vi "G#MethodTemplates_GetAttributes.vi"(0 "reference in":refnum<class "G#MethodTemplates.lvclass">, 1 "return data? (T)":bool=TRUE, 5 "error in (no error)":errorcluster) -> (14 "reference out":refnum<class "G#MethodTemplates.lvclass">, 15 "attributes ref":T2, 16 "attributes":T1, 19 "error out":errorcluster)   [LabVIEW 2020, in "G#MethodTemplates.lvclass"]
doc: "Returns a reference and if wanted the actual data values of the attributes. This method is used by the subclasses to access parent attributes."
uses:
  G#MethodTemplates.lvclass
  ObjectAttributesRef.ctl
  protected/ObjectAttributes.ctl
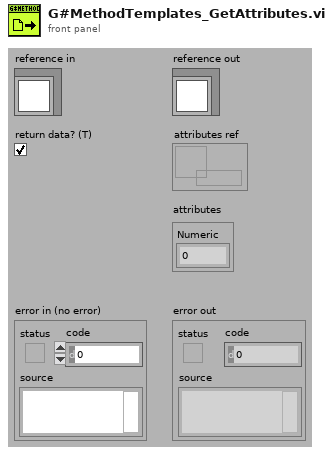
[diagram p1: front panel]
types:
  T1 = typedef "G#MethodTemplates.lvclass/ObjectAttributes.ctl" = cluster{"Numeric":dbl}
  T2 = typedef "G#MethodTemplates.lvclass/ObjectAttributesRef.ctl" = refnum<data-value>
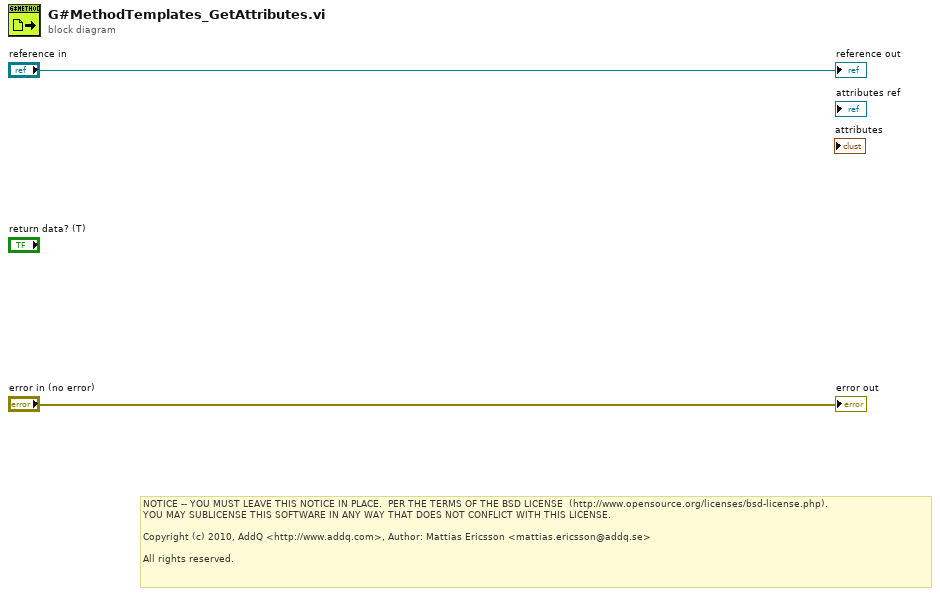
[diagram p0: block diagram]
diagram:
  # "NOTICE -- YOU MUST LEAVE THIS NOTICE IN PLACE.  PER THE TERMS OF THE BSD LICENSE  (http://www.opensource.org/licenses/bsd-license.php).\nYOU MAY SUBLICENSE THIS SOFTWARE IN ANY WAY THAT DOES NOT CONFLICT WITH THIS LICENSE.\n\nCopyright (c) 2010, AddQ <http://www.addq.com>, Author: Mattias Ericsson <mattias.ericsson@addq.se>\n\nAll rights reserved."
  "error out" <- "error in (no error)"
  "reference out" <- "reference in"
